vi "PullBack.vi"(5 "dog shifter timeout (s)":i32, 6 "Output":dbl=1.0 format="%#_13g", 7 "winch timeout (s)":i32, 8 "error in (no error)":errorcluster, 10 "WinchControlDevRef":T1={"DeviceStatus"={"status"=FALSE, "code"=0, "source"=""}, "Type"=enum."PWM", "PWM"={"Controller"=enum."Controller 1", "PWM Channel"=enum."Invalid", "DeadBand"={"Name"="", "maxPositivePwm"=0, "minPositivePwm"=0, "centerPwm"=0, "maxNegativePwm"=0, "minNegativePwm"=0, "angularRange"=0}}, "CAN"={"Device Number"=0, "Control Mode"=enum."Percent VBus", "Semaphore"=refnum, "Max Vout"=12.0}, "Invert"=FALSE, "TransformRef"=refnum, "InvTransformRef"=refnum}, 11 "LaunchReleaseMotorControlDevRef":T1={"DeviceStatus"={"status"=FALSE, "code"=0, "source"=""}, "Type"=enum."PWM", "PWM"={"Controller"=enum."Controller 1", "PWM Channel"=enum."Invalid", "DeadBand"={"Name"="", "maxPositivePwm"=0, "minPositivePwm"=0, "centerPwm"=0, "maxNegativePwm"=0, "minNegativePwm"=0, "angularRange"=0}}, "CAN"={"Device Number"=0, "Control Mode"=enum."Percent VBus", "Semaphore"=refnum, "Max Vout"=12.0}, "Invert"=FALSE, "TransformRef"=refnum, "InvTransformRef"=refnum}) -> (0 "error out":errorcluster, 2 "WinchControlDevRef":T1={"DeviceStatus"={"status"=FALSE, "code"=0, "source"=""}, "Type"=enum."PWM", "PWM"={"Controller"=enum."Controller 1", "PWM Channel"=enum."Invalid", "DeadBand"={"Name"="", "maxPositivePwm"=0, "minPositivePwm"=0, "centerPwm"=0, "maxNegativePwm"=0, "minNegativePwm"=0, "angularRange"=0}}, "CAN"={"Device Number"=0, "Control Mode"=enum."Percent VBus", "Semaphore"=refnum, "Max Vout"=12.0}, "Invert"=FALSE, "TransformRef"=refnum, "InvTransformRef"=refnum}, 3 "LaunchReleaseMotorControlDevRef":T1={"DeviceStatus"={"status"=FALSE, "code"=0, "source"=""}, "Type"=enum."PWM", "PWM"={"Controller"=enum."Controller 1", "PWM Channel"=enum."Invalid", "DeadBand"={"Name"="", "maxPositivePwm"=0, "minPositivePwm"=0, "centerPwm"=0, "maxNegativePwm"=0, "minNegativePwm"=0, "angularRange"=0}}, "CAN"={"Device Number"=0, "Control Mode"=enum."Percent VBus", "Semaphore"=refnum, "Max Vout"=12.0}, "Invert"=FALSE, "TransformRef"=refnum, "InvTransformRef"=refnum})   [LabVIEW 2014]
uses:
  <vilib>/Rock Robotics/WPI/MotorControl/WPI_MotorControlDeviceRef.ctl
  <vilib>/Rock Robotics/SystemInterfaces/Typedef/FPGA_TypedefDigitalModule.ctl
  <vilib>/Rock Robotics/SystemInterfaces/DIO/FPGA_DIOPWMChannel.ctl
  <vilib>/Rock Robotics/WPI/PWM/WPI_PWMDeadband.ctl
  <vilib>/Rock Robotics/WPI/CAN/Jaguar/SubVIs/WPI_CANJaguar_ControlMode.ctl
  <vilib>/Rock Robotics/WPI/PWM/WPI_PWMTransform_ConPane.ctl
  <vilib>/Rock Robotics/WPI/CAN/Jaguar/SubVIs/WPI_CANJaguar_StatusSelect.ctl
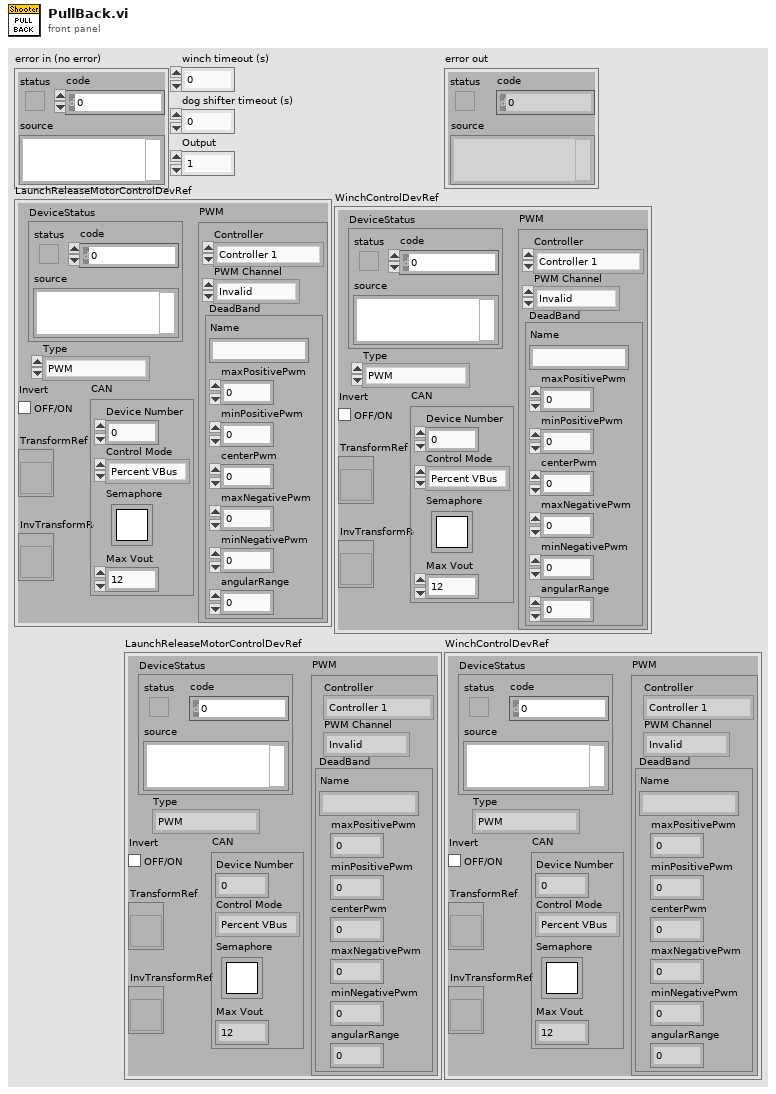
[diagram p1: front panel]
types:
  T1 = typedef "WPI_MotorControlDeviceRef.ctl" = cluster{"DeviceStatus":errorcluster, "Type":enum16{"PWM", "CAN"}, "PWM":cluster{"Controller":T2, "PWM Channel":T3, "DeadBand":T4}, "CAN":cluster{"Device Number":u8, "Control Mode":T5, "Semaphore":T6, "Max Vout":dbl}, "Invert":bool, "TransformRef":T7, "InvTransformRef":T7}
  T2 = typedef "FPGA_TypedefDigitalModule.ctl" = enum16{"Controller 1"}
  T3 = typedef "FPGA_DIOPWMChannel.ctl" = enum8{"PWM 0", "PWM 1", "PWM 2", "PWM 3", "PWM 4", "PWM 5", "PWM 6", "PWM 7", "PWM 8", "PWM 9", "PWM MXP 0", "PWM MXP 1", "PWM MXP 2", "PWM MXP 3", "PWM MXP 4", "PWM MXP 5", "PWM MXP 6", "PWM MXP 7", "PWM MXP 8", "PWM MXP 9", "Invalid"}
  T4 = typedef "WPI_PWMDeadband.ctl" = cluster{"Name":string, "maxPositivePwm":i32, "minPositivePwm":i32, "centerPwm":i32, "maxNegativePwm":i32, "minNegativePwm":i32, "angularRange":u16}
  T5 = typedef "WPI_CANJaguar_ControlMode.ctl" = enum8{"Percent VBus", "Current", "Speed", "Position", "Voltage"}
  T6 = typedef "Semaphore RefNum" = refnum<k1>
  T7 = typedef "WPI_PWMTransform_ConPane.ctl" = refnum<vi>
  T8 = typedef "WPI_CANJaguar_StatusSelect.ctl" = enum16{"Output Percent VBus", "Output Voltage", "Bus Voltage", "Current", "Temperature", "Position", "Speed", "Limit Switches", "Faults", "Fault Counters", "Power Cycle"}
  T9 = typedef "WPI_CANJaguar_Status.ctl" = cluster{"Output Percent VBus":dbl, "Output Voltage":dbl, "Bus Voltage":dbl, "Current":dbl, "Temperature":dbl, "Position":dbl, "Speed":dbl, "Limits":cluster{"Forward Limit":bool, "Reverse Limit":bool, "Forward Soft Limit":bool, "Reverse Soft Limit":bool, "Sticky Forward Limit":bool, "Sticky Reverse Limit":bool, "Sticky Forward Soft Limit":bool, "Sticky Reverse Soft Limit":bool}, "Faults":cluster{"Current Fault":bool, "Temperature Fault":bool, "Bus Voltage Fault":bool, "Gate Driver Fault":bool, "Comm Fault":bool}, "Fault Counters":cluster{"Current Faults":u8, "Temperature Faults":u8, "Bus Voltage Faults":u8, "Gate Driver Faults":u8, "Comm Faults":u8, "CAN Status":u8, "CAN RX Errors":u8, "CAN TX Errors":u8}, "Power Cycle":bool}
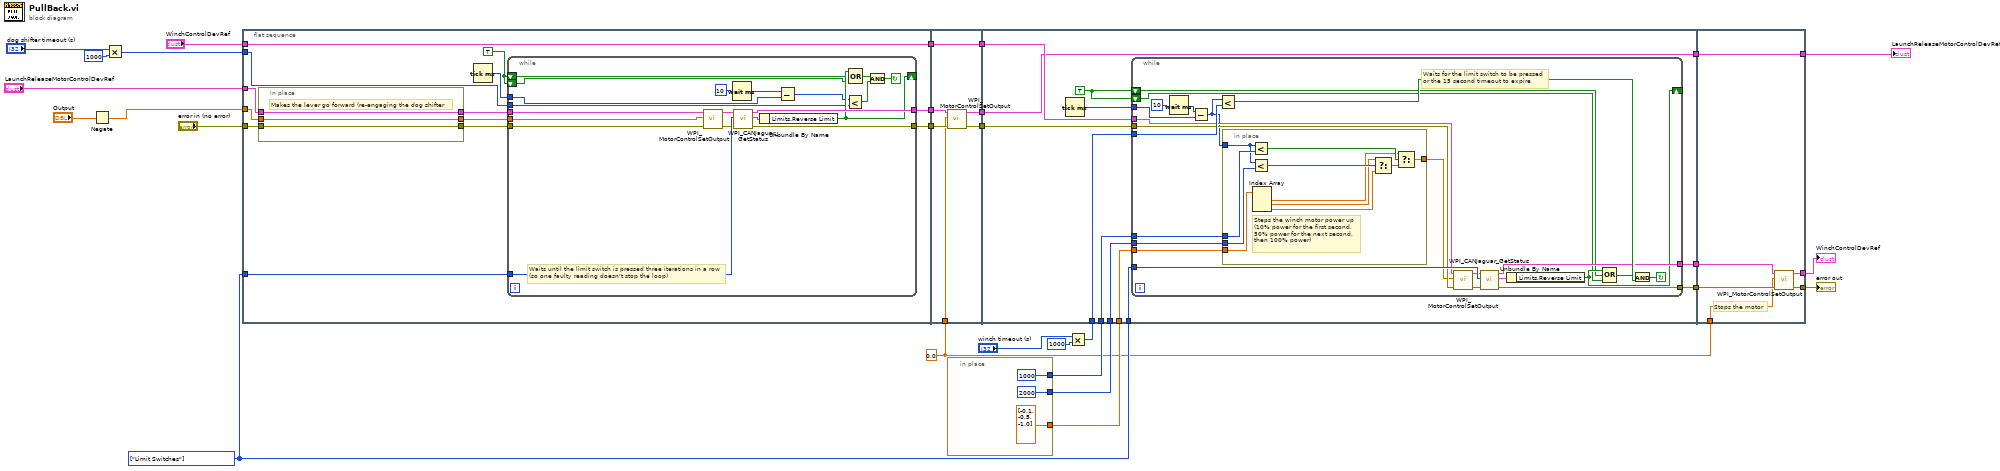
[diagram p0: block diagram]
diagram:
  w13 = 0.0 ("Output")
  w18 = T8[] [enum."Limit Switches"] items=["Output Percent VBus", "Output Voltage", "Bus Voltage", "Current", "Temperature", "Position", "Speed", "Limit Switches", "Faults", "Fault Counters", "Power Cycle"] ("Status Select")
  n1 = Negate(x="Output") -> (-x=w8:dbl)
  n2 = Multiply(x="dog shifter timeout (s)", y=1000) -> (x*y=w12:i32)
  n3 = flat-sequence {
    tunnel: [w29] -> w16
    tunnel: w8 -> [w41]
    tunnel: w18 -> [w36]
    tunnel: [w32] -> w14
    tunnel: w12 -> [w34]
    tunnel: [w33] -> w9
    tunnel: "LaunchReleaseMotorControlDevRef" -> [w31]
    tunnel: "error in (no error)" -> [w30]
    tunnel: "WinchControlDevRef" -> [w29]
    tunnel: [w68] -> w17
    tunnel: w16 -> [w70]
    tunnel: [w70] -> w15
    tunnel: w14 -> [w67]
    tunnel: w13 -> [w66]
    tunnel: w9 -> [w69]
    tunnel: [w65] -> w2
    tunnel: w17 -> [w76]
    tunnel: [w79] -> w28
    tunnel: [w78] -> w27
    tunnel: w18 -> [w82]
    tunnel: w15 -> [w77]
    tunnel: w23 -> [w80]
    tunnel: w22 -> [w75]
    tunnel: w21 -> [w74]
    tunnel: w20 -> [w73]
    tunnel: [w71] -> w3
    tunnel: w2 -> [w71]
    tunnel: w28 -> [w122]
    tunnel: w27 -> [w121]
    tunnel: [w120] -> w26
    tunnel: w13 -> [w119]
    tunnel: [w118] -> w4
    tunnel: [w117] -> w1
    tunnel: w3 -> [w117]
    frame #0 {
      w40 = TRUE
      n4 = in-place {
        in-place-border: w31 -> [w63]
        in-place-border: w30 -> [w64]
        in-place-border: w41 -> [w62]
        in-place-border: [w64] -> w38
        in-place-border: [w63] -> w39
        in-place-border: [w62] -> w37
        # "Makes the lever go forward (re-engaging the dog shifter"
      }
      n5 = Tick Count (ms)() -> (millisecond timer value=w35:u32)
      n6 = while {
        tunnel: w36 -> [w59]
        tunnel: [w58] -> w33
        shift-right: [w57] -> _
        shift-left: w40 -> [w56]
        shift-left: w40 -> [w55]
        tunnel: [w60] -> w32
        tunnel: w35 -> [w50]
        tunnel: w34 -> [w47]
        tunnel: w38 -> [w45]
        tunnel: w39 -> [w44]
        tunnel: w37 -> [w43]
        stop <- w49 continue-if-true
        # "Waits until the limit switch is pressed three iterations in a row\n(so one faulty reading doesn't stop the loop)"
        n7 = call <vilib>:"WPI_MotorControlSetOutput.vi"("error in (no error)"=w45, "Output"=w43, "MotorControlDevRef"=w44) -> ("error out"=w46:errorcluster, "MotorControlDevRef"=w42:T1)  [unwired: 6 in, 1 out]
        n8 = Wait (ms)(milliseconds to wait=u32 10) -> (millisecond timer value=w52:u32)
        n9 = call <vilib>:"WPI_CANJaguar_GetStatus.vi"("error in (no error)"=w46, "Status Select"=w59, "CAN Jaguar Ref"=w42) -> ("error out"=w58:errorcluster, "Status"=w61:T9, "CAN Jaguar Ref Out"=w60:T1)  [unwired: 6 in]
        n10 = Unbundle By Name(w61) -> ("Limits.Reverse Limit"=w57:bool)
        n11 = Subtract(x=w52, y=w50) -> (x-y=w53:u32)
        n12 = Less?(x=w53, y=w47) -> (x < y?=w48:bool)
        n13 = Compound Arithmetic op=OR(w57, w56, w55) -> (w54:bool)
        n14 = And(x=w54, y=w48) -> (x .and. y?=w49:bool)
      }
    }
    frame #1 {
      n15 = call <vilib>:"WPI_MotorControlSetOutput.vi"("error in (no error)"=w69, "Output"=w66, "MotorControlDevRef"=w67) -> ("error out"=w68:errorcluster, "MotorControlDevRef"=w65:T1)  [unwired: 6 in, 1 out]
    }
    frame #2 {
      w72 = TRUE ("Reverse Limit")
      n16 = Tick Count (ms)() -> (millisecond timer value=w81:u32)
      n17 = while {
        tunnel: w82 -> [w103]
        tunnel: w81 -> [w100]
        tunnel: w80 -> [w99]
        tunnel: w76 -> [w92]
        tunnel: [w97] -> w79
        tunnel: w77 -> [w93]
        tunnel: [w96] -> w78
        tunnel: w75 -> [w91]
        tunnel: w74 -> [w89]
        tunnel: w73 -> [w87]
        shift-right: [w86] -> _
        shift-left: w72 -> [w85]
        shift-left: w72 -> [w84]
        stop <- w102 continue-if-true
        # "Waits for the limit switch to be pressed\nor the 15 second timeout to expire"
        n18 = Wait (ms)(milliseconds to wait=u32 10) -> (millisecond timer value=w98:u32)
        n19 = Subtract(x=w98, y=w100) -> (x-y=w90:u32)
        n20 = Less?(x=w90, y=w99) -> (x < y?=w101:bool)
        n21 = in-place {
          in-place-border: w91 -> [w116]
          in-place-border: w90 -> [w114]
          in-place-border: w89 -> [w113]
          in-place-border: [w111] -> w88
          in-place-border: w87 -> [w109]
          # "Steps the winch motor power up\n(10% power for the first second,\n50% power for the next second,\nthen 100% power)"
          n22 = Less?(x=w114, y=w116) -> (x < y?=w115:bool)
          n23 = Less?(x=w114, y=w113) -> (x < y?=w110:bool)
          n24 = Index Array(array=w109) -> (element #1=w108:dbl, element #2=w107:dbl, element #3=w106:dbl)  [unwired: 3 in]
          n25 = Select(t=w107, s=w110, f=w106) -> (s? t:f=w112:dbl)
          n26 = Select(t=w108, s=w115, f=w112) -> (s? t:f=w111:dbl)
        }
        n27 = call <vilib>:"WPI_MotorControlSetOutput.vi"("error in (no error)"=w92, "Output"=w88, "MotorControlDevRef"=w93) -> ("error out"=w95:errorcluster, "MotorControlDevRef"=w94:T1)  [unwired: 6 in, 1 out]
        n28 = call <vilib>:"WPI_CANJaguar_GetStatus.vi"("error in (no error)"=w95, "Status Select"=w103, "CAN Jaguar Ref"=w94) -> ("error out"=w97:errorcluster, "Status"=w105:T9, "CAN Jaguar Ref Out"=w96:T1)  [unwired: 6 in]
        n29 = Unbundle By Name(w105) -> ("Limits.Reverse Limit"=w86:bool)
        n30 = Compound Arithmetic op=OR(w86, w85, w84) -> (w83:bool)
        n31 = And(x=w83, y=w101) -> (x .and. y?=w102:bool)
      }
    }
    frame #3 {
      # "Stops the motor"
      n32 = call <vilib>:"WPI_MotorControlSetOutput.vi"("error in (no error)"=w122, "Output"=w119, "MotorControlDevRef"=w121) -> ("error out"=w120:errorcluster, "MotorControlDevRef"=w118:T1)  [unwired: 6 in, 1 out]
    }
  }
  n33 = in-place {
    in-place-border: [u32 1000 ("y")] -> w22
    in-place-border: [u32 2000 ("y")] -> w21
    in-place-border: [dbl[] [-0.1, -0.5, -1.0]] -> w20
  }
  n34 = Multiply(x="winch timeout (s)", y=1000) -> (x*y=w23:i32)
  "error out" <- w26
  "WinchControlDevRef" <- w4
  "LaunchReleaseMotorControlDevRef" <- w1
